vi "GlueSideUp.vi"() -> ()   [LabVIEW 2015]
uses:
  GlobalPath.vi
  GlobalData.vi
  GlobalVi.vi
panel:
  in  "ptfe 10":bool caption="Repeat the same procedure one more time to ensure that the glue is perfectly plane with respect to the PCB surface (solo sul O-ring)"
  in  "ptfe 8":bool caption="Remove the excess glue using a small spatula"
  in  "ptfe 7":bool caption="Close the gap with Araldite 2011 glue using a thin syringe (coprire anche la parte di coverlay meta')"
  out "PanelName":string
  in  "DONE ALL ?":bool
  in  "ptfe 5":bool caption="Wait 24h for the glue to cure"
  # "1. PCB gap closing side up"
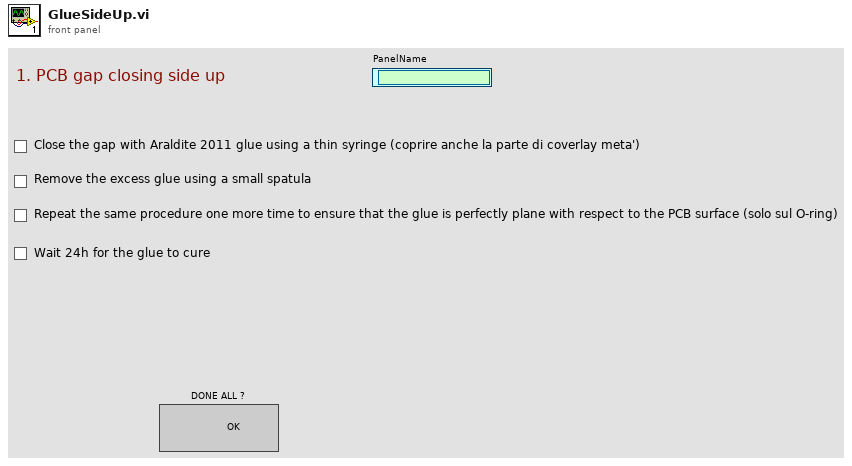
[diagram p1: front panel]
types:
  T1 = enum16{"open", "replace", "create", "open or create", "replace or create", "replace or create with confirmation"}
  T2 = enum32{"Bad", "Idle", "Run top level", "Running"}
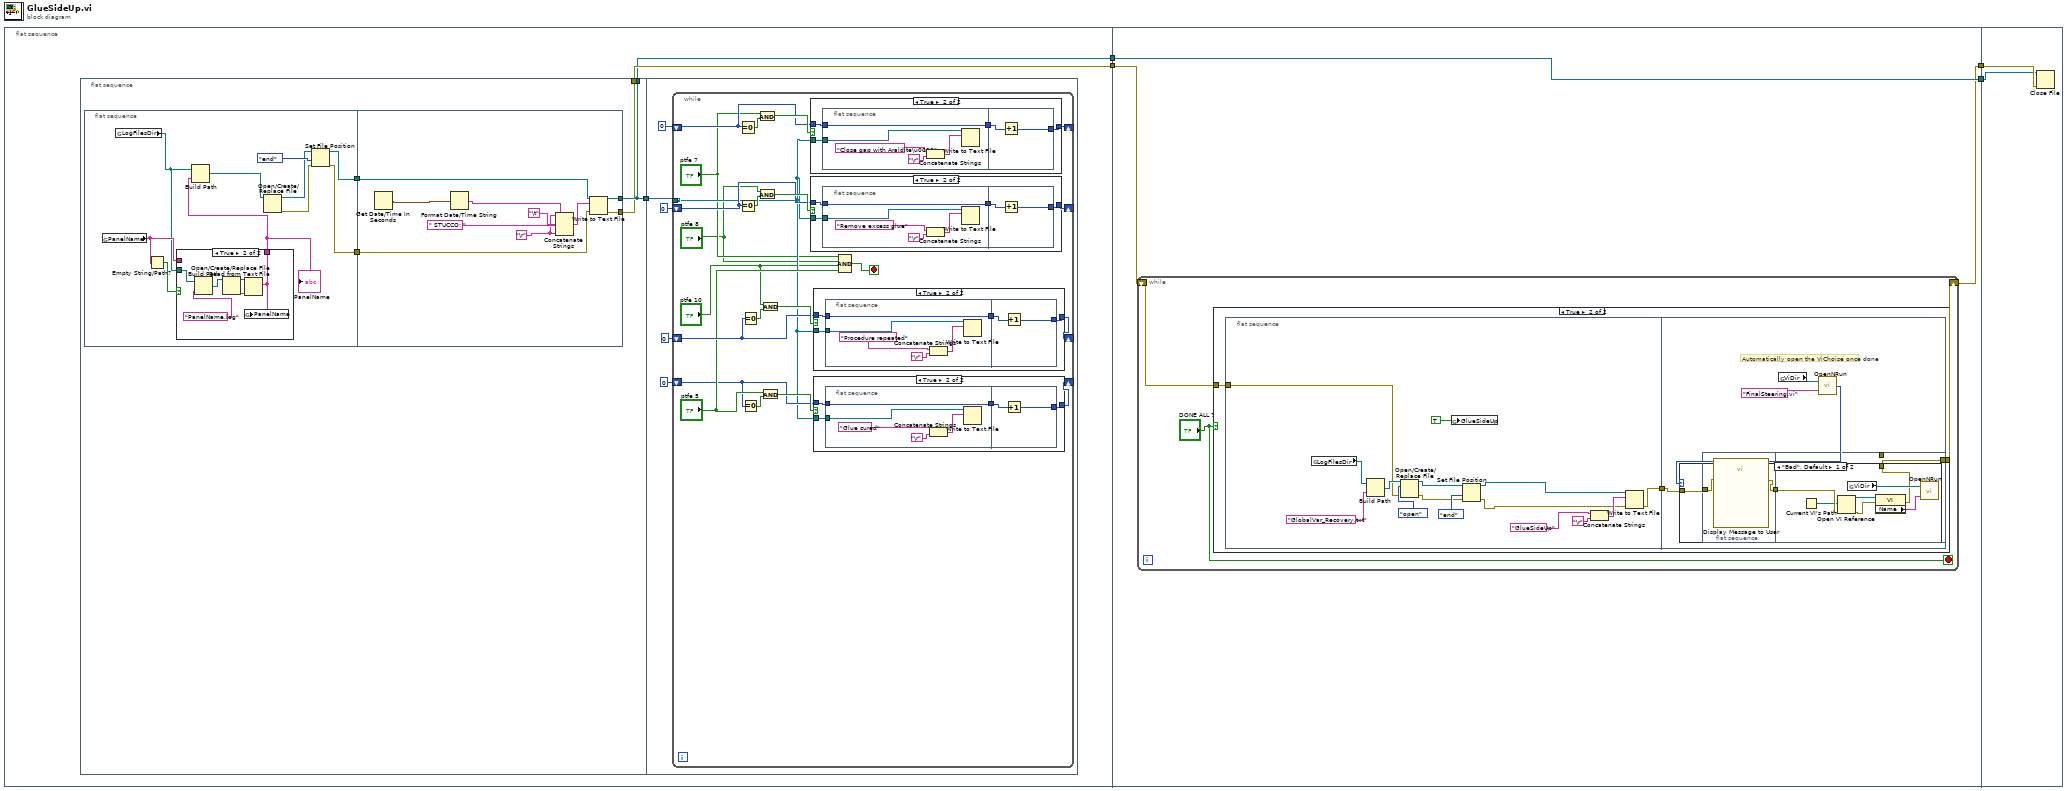
[diagram p0: block diagram]
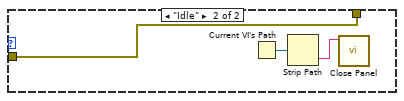
[diagram p8: hidden frame]
diagram:
  n1 = flat-sequence {
    tunnel: [w6] -> w3
    tunnel: [w5] -> w2
    tunnel: [w115] -> w4
    tunnel: w3 -> [w114]
    tunnel: w2 -> [w116]
    tunnel: [w116] -> w1
    tunnel: w4 -> [w160]
    tunnel: w1 -> [w159]
    frame #0 {
      n2 = flat-sequence {
        tunnel: [w10] -> w7
        tunnel: [w10] -> w5
        tunnel: [w9] -> w6
        tunnel: w7 -> [w43]
        frame #0 {
          n3 = flat-sequence {
            tunnel: [w16] -> w11
            tunnel: [w18] -> w8
            tunnel: w11 -> [w34]
            tunnel: [w33] -> w10
            tunnel: [w32] -> w9
            tunnel: w8 -> [w31]
            frame #0 {
              n4 = global read "GlobalData.vi" "PanelName"() -> (w15:string)
              n5 = global read "GlobalPath.vi" "LogFilesDir"() -> (w12:path)
              n6 = Empty String/Path?(string/path=w15) -> (empty?=w14:bool)
              n7 = case shown="True" w14 {
                tunnel: w12 -> [_ w28]
                tunnel: [w22 w23] -> w13
                tunnel: w15 -> [w22 _]
                frame False {
                }
                frame True {
                  n8 = Build Path(base path=w28, name or relative path="PanelName.log") -> (appended path=w27:path)
                  n9 = Open/Create/Replace File(file path (use dialog)=w27) -> (refnum out=w24:refnum<file>, error out=w25:errorcluster)  [unwired: 5 in, 1 out]
                  n10 = Read from Text File(file (use dialog)=w24, error in=w25) -> (text=w23:string)  [unwired: 2 in, 3 out]
                  n11 = global write "GlobalData.vi" "PanelName"(w23) -> ()
                }
              }
              "PanelName" <- w13
              n12 = Build Path(base path=w12, name or relative path=w13) -> (appended path=w21:path)
              n13 = Open/Create/Replace File(file path (use dialog)=w21) -> (refnum out=w17:refnum<file>, error out=w19:errorcluster)  [unwired: 5 in, 1 out]
              n14 = Set File Position(refnum=w17, from (0:start)=enum16{"start", "end", "current"}."end", error in=w19) -> (refnum out=w16:refnum<file>, error out=w18:errorcluster)  [unwired: 1 in]
            }
            frame #1 {
              w29 = "\r"
              n15 = Get Date/Time In Seconds() -> (seconds since 1Jan1904=w30:timestamp)
              n16 = Format Date/Time String(seconds (now)=w30) -> (date/time string=w36:string)  [unwired: 2 in]
              n17 = Concatenate Strings(w29, w36, "\t", " STUCCO: ", w29) -> (w35:string)
              n18 = Write to Text File(file (use dialog)=w34, text=w35, error in=w31) -> (refnum out=w33:refnum<file>, error out=w32:errorcluster)  [unwired: 1 in, 1 out]
            }
          }
        }
        frame #1 {
          n19 = while {
            tunnel: w43 -> [w47]
            shift-right: [w61] -> _
            shift-left: 0 -> [w62]
            shift-right: [w57] -> _
            shift-left: 0 -> [w58]
            shift-right: [w53] -> _
            shift-left: 0 -> [w54]
            shift-right: [w48] -> _
            shift-left: 0 -> [w49]
            stop <- w65 stop-if-true
            n20 = Equal To 0?(x=w62) -> (x = 0?=w64:bool)
            n21 = Equal To 0?(x=w58) -> (x = 0?=w60:bool)
            n22 = Equal To 0?(x=w54) -> (x = 0?=w56:bool)
            n23 = Equal To 0?(x=w49) -> (x = 0?=w52:bool)
            n24 = And(x="ptfe 7", y=w64) -> (x .and. y?=w63:bool)
            n25 = And(x="ptfe 8", y=w60) -> (x .and. y?=w59:bool)
            n26 = And(x="ptfe 10", y=w56) -> (x .and. y?=w55:bool)
            n27 = And(x="ptfe 5", y=w52) -> (x .and. y?=w51:bool)
            n28 = case shown="True" w63 {
              tunnel: w47 -> [_ w106]
              tunnel: w62 -> [w102 w104]
              tunnel: [w102 w103] -> w61
              frame False {
              }
              frame True {
                n29 = flat-sequence {
                  tunnel: w106 -> [w109]
                  tunnel: [w108] -> w105
                  tunnel: w104 -> [w108]
                  tunnel: w105 -> [w113]
                  tunnel: [w112] -> w103
                  frame #0 {
                    n30 = Concatenate Strings("Close gap with Araldite\u0000", "\r") -> (w111:string)
                    n31 = Write to Text File(file (use dialog)=w109, text=w111) -> ()  [unwired: 2 in, 3 out]
                  }
                  frame #1 {
                    n32 = Increment(x=w113) -> (x+1=w112:i32)
                  }
                }
              }
            }
            n33 = case shown="True" w59 {
              tunnel: w47 -> [_ w94]
              tunnel: w58 -> [w90 w92]
              tunnel: [w90 w91] -> w57
              frame False {
              }
              frame True {
                n34 = flat-sequence {
                  tunnel: w94 -> [w97]
                  tunnel: [w96] -> w93
                  tunnel: w92 -> [w96]
                  tunnel: w93 -> [w101]
                  tunnel: [w100] -> w91
                  frame #0 {
                    n35 = Concatenate Strings("Remove excess glue", "\r") -> (w99:string)
                    n36 = Write to Text File(file (use dialog)=w97, text=w99) -> ()  [unwired: 2 in, 3 out]
                  }
                  frame #1 {
                    n37 = Increment(x=w101) -> (x+1=w100:i32)
                  }
                }
              }
            }
            n38 = case shown="True" w55 {
              tunnel: w47 -> [_ w82]
              tunnel: w54 -> [w78 w80]
              tunnel: [w78 w79] -> w53
              frame False {
              }
              frame True {
                n39 = flat-sequence {
                  tunnel: w82 -> [w85]
                  tunnel: [w84] -> w81
                  tunnel: w80 -> [w84]
                  tunnel: w81 -> [w89]
                  tunnel: [w88] -> w79
                  frame #0 {
                    n40 = Concatenate Strings("Procedure repeated", "\r") -> (w87:string)
                    n41 = Write to Text File(file (use dialog)=w85, text=w87) -> ()  [unwired: 2 in, 3 out]
                  }
                  frame #1 {
                    n42 = Increment(x=w89) -> (x+1=w88:i32)
                  }
                }
              }
            }
            n43 = case shown="True" w51 {
              tunnel: w47 -> [_ w70]
              tunnel: w49 -> [w66 w68]
              tunnel: [w66 w67] -> w48
              frame False {
              }
              frame True {
                n44 = flat-sequence {
                  tunnel: w70 -> [w73]
                  tunnel: [w72] -> w69
                  tunnel: w68 -> [w72]
                  tunnel: w69 -> [w77]
                  tunnel: [w76] -> w67
                  frame #0 {
                    n45 = Concatenate Strings("Glue cured", "\r") -> (w75:string)
                    n46 = Write to Text File(file (use dialog)=w73, text=w75) -> ()  [unwired: 2 in, 3 out]
                  }
                  frame #1 {
                    n47 = Increment(x=w77) -> (x+1=w76:i32)
                  }
                }
              }
            }
            n48 = Compound Arithmetic op=AND("ptfe 7", "ptfe 8", "ptfe 10", "ptfe 5") -> (w65:bool)
          }
        }
      }
    }
    frame #1 {
      n49 = while {
        shift-right: [w119] -> w115
        shift-left: w114 -> [w118]
        stop <- "DONE ALL ?" stop-if-true
        n50 = case shown="True" "DONE ALL ?" {
          tunnel: [w120 w123] -> w119
          tunnel: w118 -> [w120 w122]
          frame False {
          }
          frame True {
            n51 = flat-sequence {
              tunnel: w122 -> [w127]
              tunnel: [w126] -> w121
              tunnel: [w140] -> w123
              tunnel: w121 -> [w139]
              frame #0 {
                n52 = global read "GlobalPath.vi" "LogFilesDir"() -> (w124:path)
                n53 = Build Path(base path=w124, name or relative path="GlobalVar_Recovery.txt") -> (appended path=w136:path)
                n54 = Open/Create/Replace File(file path (use dialog)=w136, error in=w127, operation (0:open)=T1."open") -> (refnum out=w132:refnum<file>, error out=w133:errorcluster)  [unwired: 3 in, 1 out]
                n55 = global write "GlobalVi.vi" "GlueSideUp"(TRUE) -> ()
                n56 = Set File Position(refnum=w132, from (0:start)=enum16{"start", "end", "current"}."end", error in=w133) -> (refnum out=w129:refnum<file>, error out=w128:errorcluster)  [unwired: 1 in]
                n57 = Concatenate Strings("GlueSideUp", "\r") -> (w131:string)
                n58 = Write to Text File(file (use dialog)=w129, text=w131, error in=w128) -> (error out=w126:errorcluster)  [unwired: 1 in, 2 out]
              }
              frame #1 {
                # "Automatically open the ViChoise once done"
                n59 = global read "GlobalPath.vi" "ViDir"() -> (w143:path)
                n60 = call "OpenNRun.vi"("VI name"="FinalSteering.vi", "ViDirPath"=w143) -> ("Execution:State"=w142:T2)
                n61 = case shown="\"Bad\", Default" w142 {
                  tunnel: [w144 w156] -> w140
                  tunnel: w139 -> [w145 w156]
                  frame "Bad", Default {
                    n62 = flat-sequence {
                      tunnel: w145 -> [w148]
                      tunnel: [w147] -> w146
                      tunnel: w146 -> [w152]
                      tunnel: [w149] -> w144
                      frame #0 {
                        n63 = call "Display Message to User"("error in (no error)"=w148) -> ("error out"=w147:errorcluster)  [unwired: 9 in, 1 out]
                      }
                      frame #1 {
                        n64 = Current VI's Path() -> (path=w150:path)
                        n65 = Open VI Reference(vi path=w150, error in (no error)=w152) -> (vi reference=w155:refnum<vi>, error out=w154:errorcluster)  [unwired: 4 in]
                        n66 = global read "GlobalPath.vi" "ViDir"() -> (w151:path)
                        n67 = property class="VI"(reference=w155, error in=w154) -> (error out=w149:errorcluster, "Name"=w153:string)  [unwired: 1 out]
                        n68 = call "OpenNRun.vi"("VI name"=w153, "ViDirPath"=w151) -> ()  [unwired: 1 out]
                      }
                    }
                  }
                  frame "Idle" {
                    n69 = Current VI's Path() -> (path=w157:path)
                    n70 = Strip Path(path=w157) -> (name=w158:string)  [unwired: 1 out]
                    n71 = call <vilib>:"Close Panel.vi"("VI name"=w158) -> ()  [unwired: 10 in, 1 out]
                  }
                }
              }
            }
          }
        }
      }
    }
    frame #2 {
      n72 = Close File(refnum=w159, error in=w160) -> ()  [unwired: 2 out]
    }
  }
